vi "myRIO_BRig_RT_dataExp_Audio_amp__L.vi"() -> (2 "output_Audio_amp__L":i32)   [LabVIEW 2014]
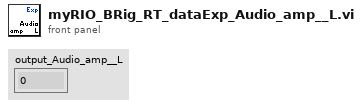
[diagram p1: front panel]
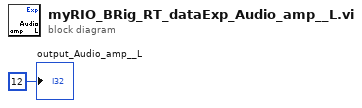
[diagram p0: block diagram]
diagram:
  "output_Audio_amp__L" <- 12 ("output_iBlock")
